vi "Measure Waveform.vi"(8 "error in":errorcluster, 9 "timeout[s]":dbl=10.0 format="%0.2f", 10 "number of samples per channel":i32=-1, 11 "task/channel":refnum<k21>="Station2_DUT1") -> (0 "error out":errorcluster, 2 "data":waveform(dbl)[](array[waveform]), 3 "task out":refnum<k21>)   [LabVIEW 2023, in "AI.lvlib"]
uses:
  AI.lvlib
  <vilib>/DAQmx/read.llb/DAQmx Read (Analog 1D Wfm NChan NSamp).vi
  <vilib>/DAQmx/miscellaneous.llb/DAQmx Fill In Error Info.vi
panel:
  out "Waveform Graph":waveform(dbl)[](graph)
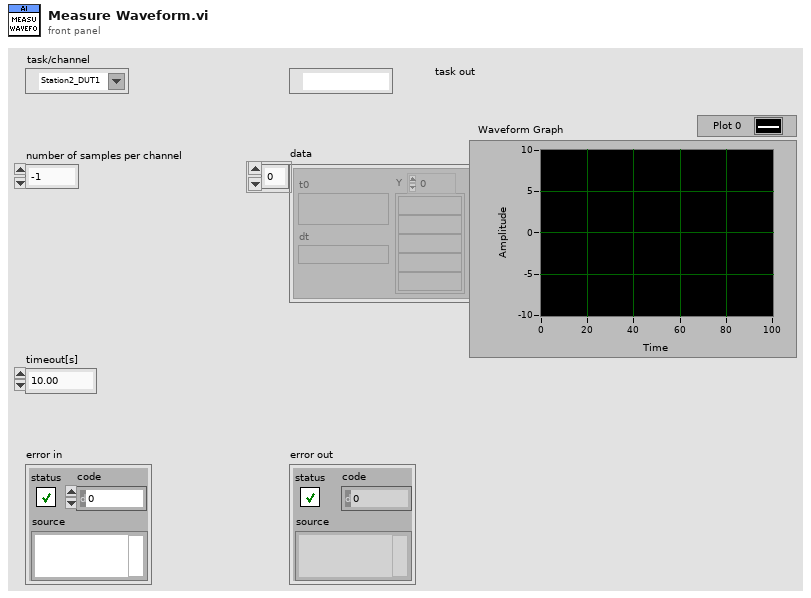
[diagram p1: front panel]
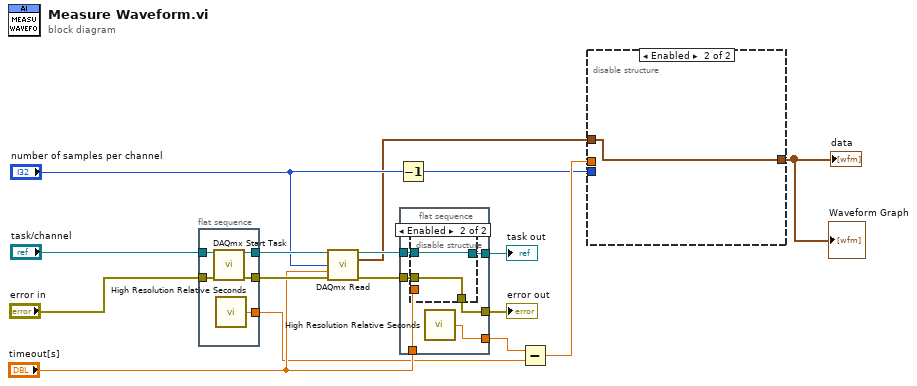
[diagram p0: block diagram]
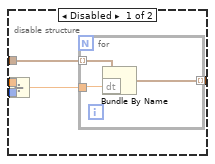
[diagram p2: hidden frame]
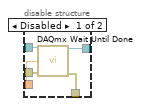
[diagram p3: hidden frame]
diagram:
  n1 = flat-sequence {
    tunnel: "error in" -> [w21]
    tunnel: [w20] -> w15
    tunnel: [w19] -> w14
    tunnel: "task/channel" -> [w18]
    tunnel: [w17] -> w6
    frame #0 {
      n2 = call <vilib>:"DAQmx Start Task.vi"("task/channels in"=w18, "error in"=w21) -> ("task out"=w20:refnum<k21>, "error out"=w19:errorcluster)  [unwired: 12 in]
      n3 = call <vilib>:"High Resolution Relative Seconds.vi"() -> ("relative seconds"=w17:dbl)
    }
  }
  n4 = call-poly <vilib>:"DAQmx Read.vi"("task/channels in"=w15, "number of samples per channel"="number of samples per channel", "timeout"="timeout[s]", "error in"=w14) -> ("task out"=w13:refnum<k21>, "data"=w4:waveform(dbl)[], "error out"=w12:errorcluster)  [unwired: 9 in]
  n5 = Decrement(x="number of samples per channel") -> (x-1=w2:i32)
  n6 = flat-sequence {
    tunnel: w13 -> [w27]
    tunnel: w12 -> [w26]
    tunnel: "timeout[s]" -> [w25]
    tunnel: [w24] -> w10
    tunnel: [w23] -> w9
    tunnel: [w22] -> w7
    frame #0 {
      n7 = disable-structure shown="Enabled" {
        disable-tunnel: w27 -> [w32 w34]
        disable-tunnel: w26 -> [w31 w33]
        disable-tunnel: w25 -> [w30 _]
        disable-tunnel: [w29 w33] -> w24
        disable-tunnel: [w28 w34] -> w23
        frame Disabled {
          n8 = call <vilib>:"DAQmx Wait Until Done.vi"("task/channels in"=w32, "timeout (sec)"=w30, "error in"=w31) -> ("task out"=w28:refnum<k21>, "error out"=w29:errorcluster)  [unwired: 11 in]
        }
        frame Enabled {
        }
      }
      n9 = call <vilib>:"High Resolution Relative Seconds.vi"() -> ("relative seconds"=w22:dbl)
    }
  }
  n10 = Subtract(x=w7, y=w6) -> (x-y=w3:dbl)
  n11 = disable-structure shown="Enabled" {
    disable-tunnel: w4 -> [w39 w43]
    disable-tunnel: w3 -> [w37 _]
    disable-tunnel: w2 -> [w36 _]
    disable-tunnel: [w35 w43] -> w1
    frame Disabled {
      n12 = Divide(x=w37, y=w36) -> (x/y=w38:dbl)
      n13 = for {
        tunnel: w39 -> [w42] mode=indexing
        tunnel: [w41] -> w35 mode=indexing
        tunnel: w38 -> [w40]
        n14 = Bundle By Name(cluster=w42, "dt"=w40) -> (w41:waveform(dbl))
      }
    }
    frame Enabled {
    }
  }
  "data" <- w1
  "Waveform Graph" <- w1
  "task out" <- w9
  "error out" <- w10
